vi "Write Custom Char.vi"(8 "error in (no error)":errorcluster, 9 "Char":bool[][](array[boolean])=[[FALSE, FALSE, FALSE, FALSE, FALSE], [FALSE, FALSE, FALSE, FALSE, FALSE], [FALSE, FALSE, FALSE, FALSE, FALSE], [FALSE, FALSE, FALSE, FALSE, FALSE], [FALSE, FALSE, FALSE, FALSE, FALSE], [FALSE, FALSE, FALSE, FALSE, FALSE], [FALSE, FALSE, FALSE, FALSE, FALSE], [FALSE, FALSE, FALSE, FALSE, FALSE]], 11 "Grove I2C Matrix LED in":refnum<class "Grove I2C Matrix LED Driver.lvclass">) -> (0 "error out":errorcluster, 3 "Grove I2C Matrix LED out":refnum<class "Grove I2C Matrix LED Driver.lvclass">)   [LabVIEW 2020, in "CTI-Peripheral.lvlib" / "Grove I2C Matrix LED Driver.lvclass"]
uses:
  Grove I2C Matrix LED Driver.lvclass
  Grove I2C Matrix LED Driver.lvclass/Grove I2C Matrix LED Driver.ctl
  CTI/I2C Connection/I2C Connection.lvclass/I2C Connection.ctl
  CTI/Session/I2C Write Data.vi
  CTI/I2C Connection/I2C Connection.lvclass
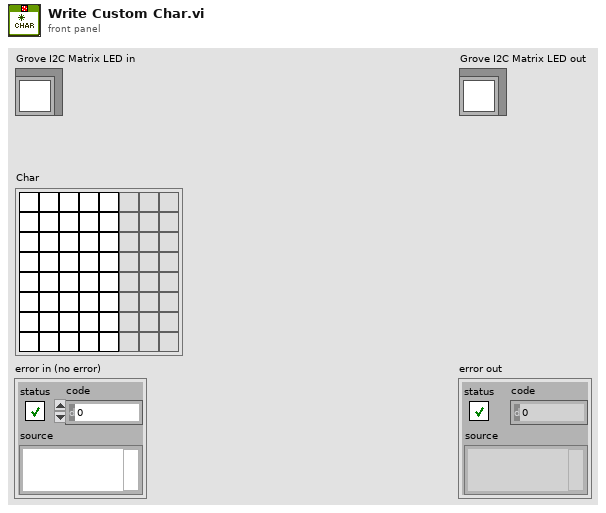
[diagram p1: front panel]
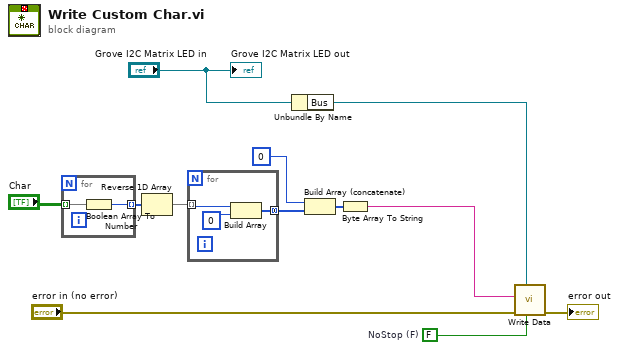
[diagram p0: block diagram]
diagram:
  w10 = FALSE  # NoStop (F)
  n1 = for {
    tunnel: "Char" -> [w14] mode=indexing
    tunnel: [w13] -> w12 mode=indexing
    n2 = Boolean Array To Number(Boolean array=w14) -> (number=w13:u32)
  }
  n3 = Reverse 1D Array(array=w12) -> (reversed array=w5:u32[])
  n4 = for {
    tunnel: w5 -> [w17] mode=indexing
    tunnel: [w15] -> w4 mode=concatenating
    n5 = Build Array(w17, u8 0 ("Value")) -> (w15:u32[])
  }
  n6 = Unbundle By Name("Grove I2C Matrix LED in") -> ("Bus"=w2:refnum<class "I2C Connection.lvclass">)
  n7 = Build Array (concatenate)(u8 0 ("Value"), w4) -> (w7:u32[])
  n8 = Byte Array To String(unsigned byte array=w7) -> (string=w1:string)
  n9 = call "Write Data.vi"("NoStop (F)"=w10, "I2C Connection"=w2, "error in (no error)"="error in (no error)", "Data"=w1) -> ("error out"=→"error out":errorcluster)  [unwired: 7 in]
  "Grove I2C Matrix LED out" <- "Grove I2C Matrix LED in"
